vi "CIF_CIPC_String_Tag Update Test Cases.vi"() -> (0 "error out":errorcluster, 2 "status":string, 3 "pass":bool)   [LabVIEW 2021]
uses:
  CIFChannels/Typedef/Direction.ctl
  CIF_CIPC_Chn_String.lvclass
  D:/dev/Packages/CIF_Channels_Core/src/CIFChannels/CIFChannels.lvclass
  ChannelCommon/typedef/New FIFO Instance Response.ctl
  ChannelCommon/typedef/New FIFO Config.ctl
  ChannelCommon/typedef/FIFO Flags.ctl
  ChannelCommon/Utilities/Flatten FIFO Config.vi
  ChannelCommon/Utilities/Flatten FIFO Flags.vi
  <vilib>/CIF Foundation/CIF Utilities/DataTypes/Flatten Unflatten/Flatten U64.vi
  CIFChannels/CIFChannels.lvclass
  ChannelCommon/ChannelCommon.lvlib
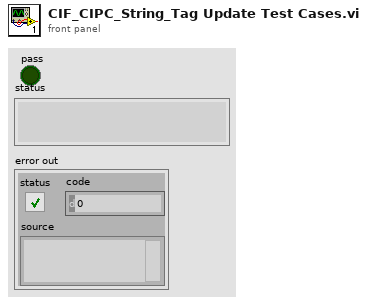
[diagram p1: front panel]
types:
  T1 = typedef "CIFChannels.lvclass/Direction.ctl" = enum16{"Publisher", "Subscriber"}
  T2 = typedef "ChannelCommon.lvlib/New FIFO Instance Response.ctl" = cluster{"Publisher":string, "Custom Data":u8[]}
  T3 = typedef "ChannelCommon.lvlib/New FIFO Config.ctl" = cluster{"Max Bytes/Msg":u64, "Max Msg/FIFO":u64, "FIFO Flags":T4}
  T4 = typedef "ChannelCommon.lvlib/FIFO Flags.ctl" = cluster{"Backpressure":bool}
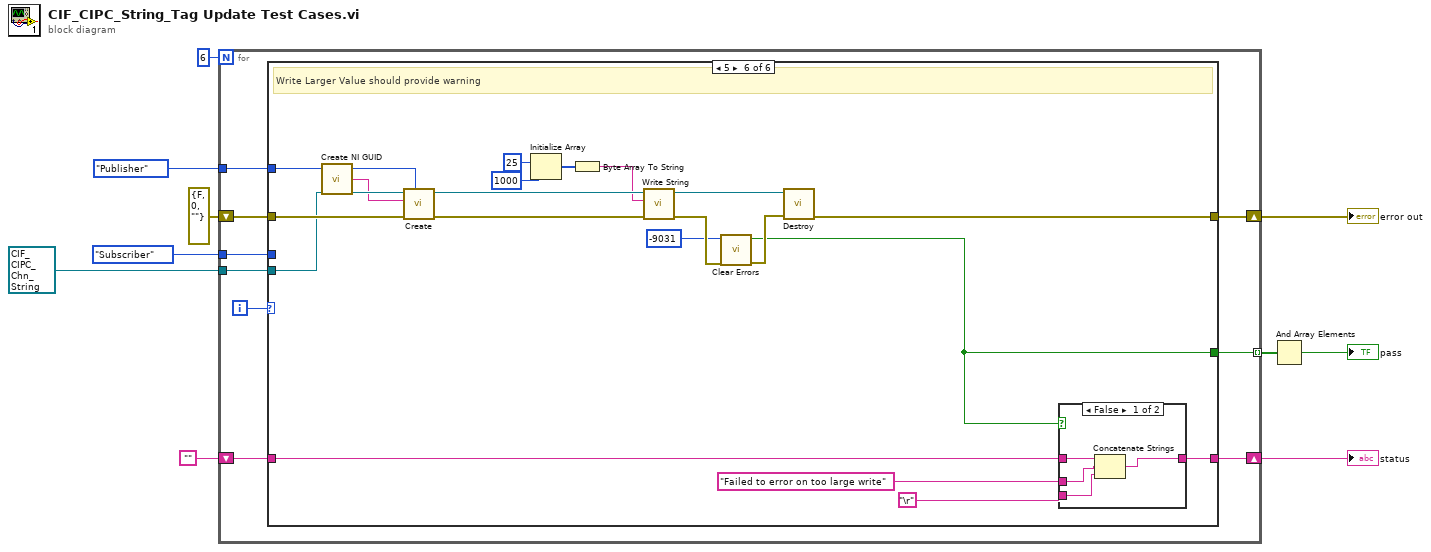
[diagram p0: block diagram]
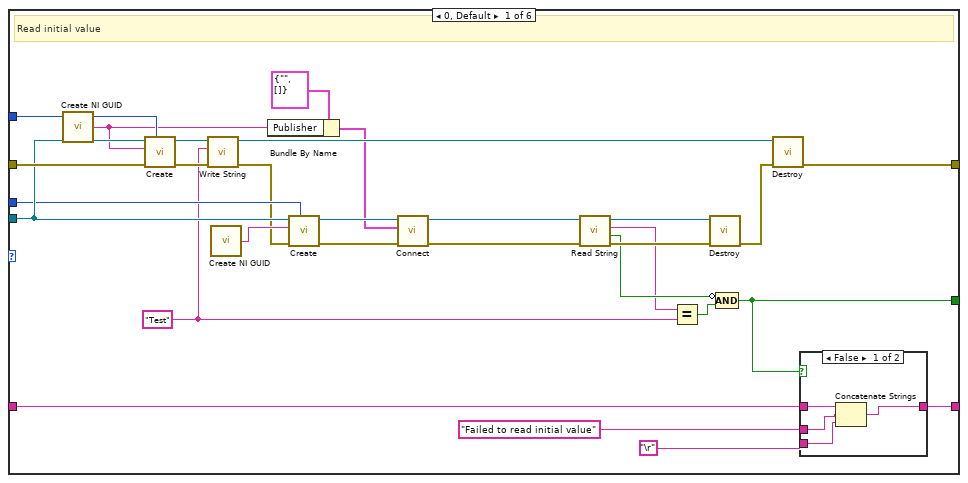
[diagram p2: hidden frame]
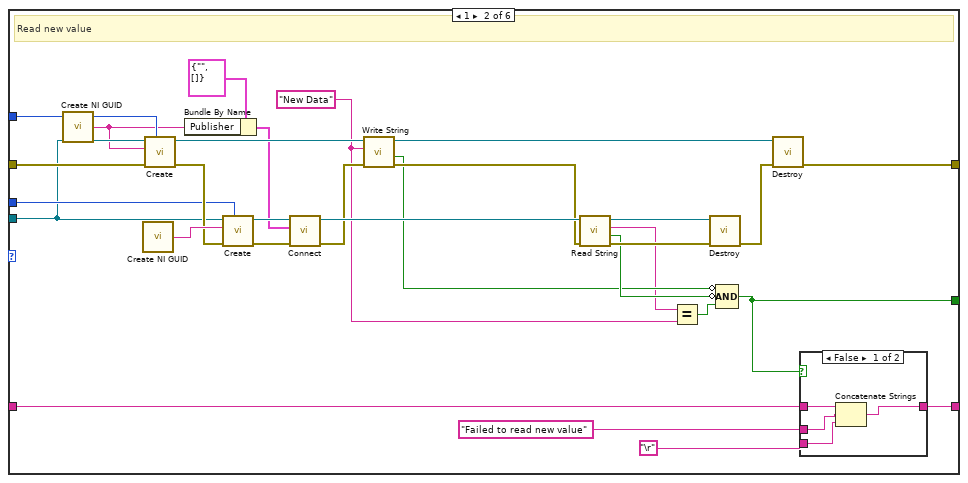
[diagram p4: hidden frame]
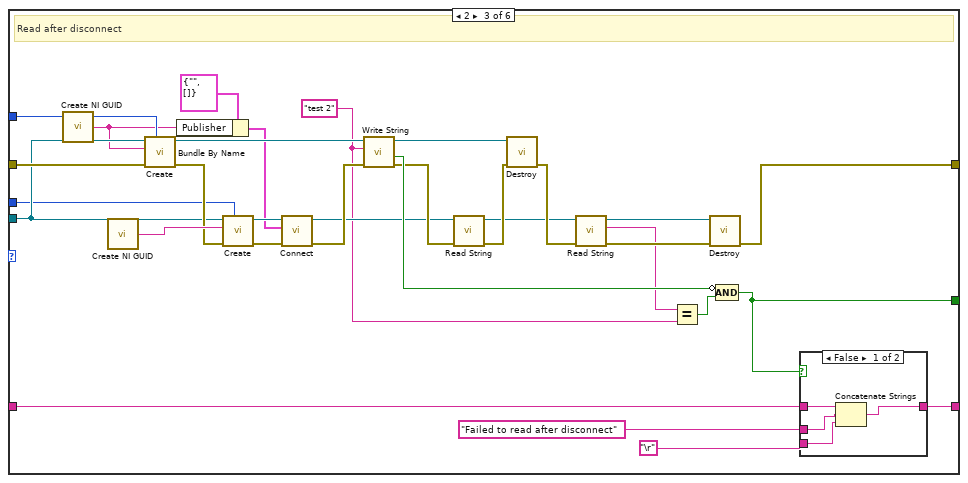
[diagram p6: hidden frame]
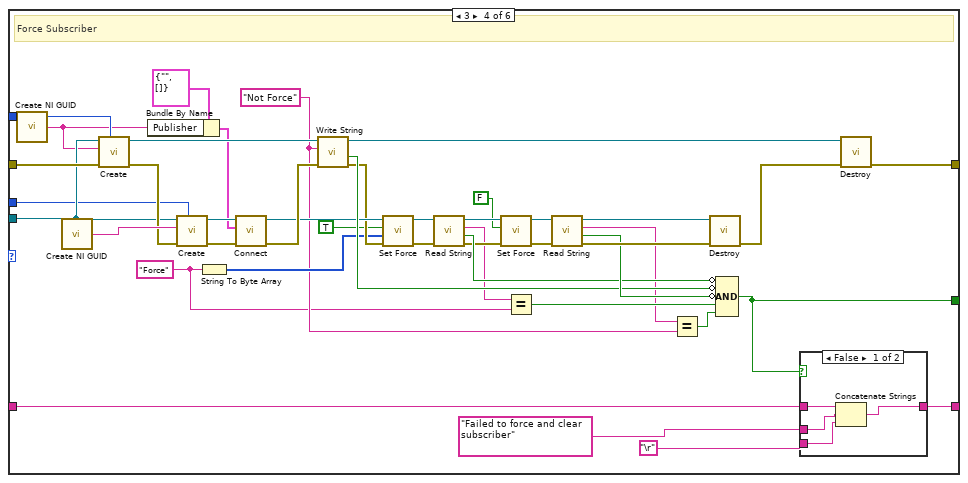
[diagram p8: hidden frame]
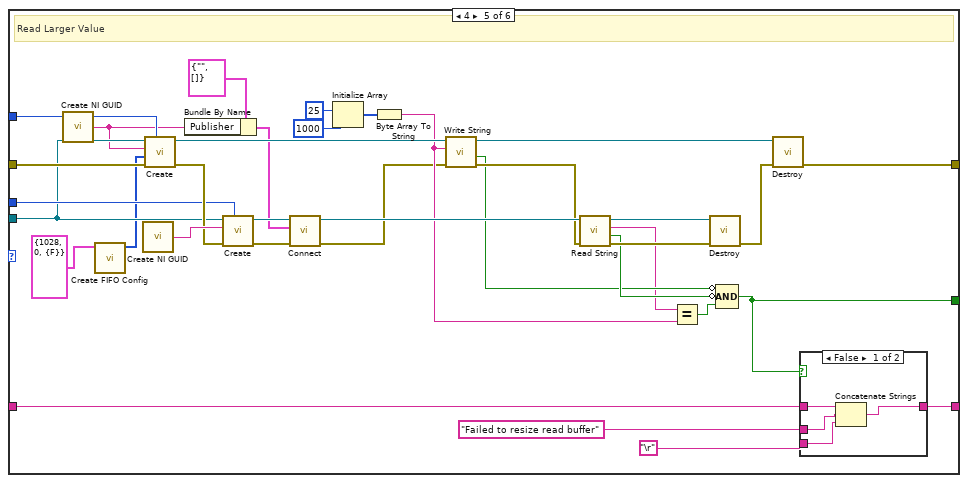
[diagram p10: hidden frame]
diagram:
  n1 = for {
    N: 6 -> [_]
    tunnel: [w19] -> w10 mode=indexing
    shift-right: [w17] -> w5
    shift-left: errorcluster {"status"=FALSE, "code"=0, "source"=""} ("error out") -> [w18]
    shift-right: [w14] -> w6
    shift-left: "" -> [w15]
    tunnel: refnum<class "CIF_CIPC_Chn_String.lvclass"> refnum ("CIF_CIPC_Chn_String.lvclass") -> [w13]
    tunnel: Direction."Publisher" ("Direction") -> [w12]
    tunnel: Direction."Subscriber" ("Direction") -> [w11]
    i -> [w16]
    n2 = case shown="5" w16 {
      tunnel: [w33 w68 w111 w158 w192 w213] -> w19
      tunnel: w18 -> [w44 w79 w115 w163 w203 w228]
      tunnel: [w35 w70 w105 w132 w194 w227] -> w17
      tunnel: w15 -> [w48 w83 w119 w167 w207 w232]
      tunnel: [w47 w82 w118 w166 w206 w231] -> w14
      tunnel: w13 -> [w30 w59 w100 w150 w184 w223]
      tunnel: w12 -> [w31 w61 w99 w149 w186 w224]
      tunnel: w11 -> [w29 w60 w98 w148 w185 _]
      frame 0, Default {
        w21 = "Test"
        # "Read initial value"
        n3 = call <vilib>:"Create NI GUID.vi"() -> ("NI GUID"=w23:string)
        n4 = call-dynamic "Create.vi"("Direction"=w31, "error in (no error)"=w44, "Name"=w23, "CIFTag in"=w30) -> ("error out"=w27:errorcluster, "CIFTag out"=w28:refnum<class "CIF_CIPC_Chn_String.lvclass">)  [unwired: 6 in]
        n5 = call-dynamic "Write String.vi"("error in (no error)"=w27, "Data"=w21, "CIFTag in"=w28) -> ("error out"=w25:errorcluster, "CIFTag out"=w26:refnum<class "CIF_CIPC_Chn_String.lvclass">)  [unwired: 6 in, 1 out]
        n6 = call <vilib>:"Create NI GUID.vi"() -> ("NI GUID"=w43:string)
        n7 = Bundle By Name(cluster=T2 {"Publisher"="", "Custom Data"=[]} ("Connection"), "Publisher"=w23) -> (w22:T2)
        n8 = call-dynamic "Create.vi"("Direction"=w29, "error in (no error)"=w25, "Name"=w43, "CIFTag in"=w30) -> ("error out"=w41:errorcluster, "CIFTag out"=w42:refnum<class "CIF_CIPC_Chn_String.lvclass">)  [unwired: 6 in]
        n9 = call-dynamic "Connect.vi"("error in (no error)"=w41, "Connection"=w22, "CIFTag in"=w42) -> ("error out"=w39:errorcluster, "CIFTag out"=w40:refnum<class "CIF_CIPC_Chn_String.lvclass">)  [unwired: 7 in]
        n10 = call-dynamic "Read String.vi"("error in (no error)"=w39, "CIFTag in"=w40) -> ("error out"=w37:errorcluster, "timed out?"=w32:bool, "Data"=w20:string, "CIFTag out"=w38:refnum<class "CIF_CIPC_Chn_String.lvclass">)  [unwired: 6 in]
        n11 = Equal?(x=w20, y=w21) -> (x = y?=w34:bool)
        n12 = call-dynamic "Destroy.vi"("error in (no error)"=w37, "CIFTag in"=w38) -> ("error out"=w36:errorcluster)  [unwired: 8 in, 1 out]
        n13 = Compound Arithmetic op=AND(invert w32, w34) -> (w33:bool)
        n14 = call-dynamic "Destroy.vi"("error in (no error)"=w36, "CIFTag in"=w26) -> ("error out"=w35:errorcluster)  [unwired: 8 in, 1 out]
        n15 = case shown="False" w33 {
          tunnel: w48 -> [w52 w53]
          tunnel: [w49 w53] -> w47
          tunnel: "Failed to read initial value" -> [w51 _]
          tunnel: "\r" -> [w50 _]
          frame False {
            n16 = Concatenate Strings(w52, w51, w50) -> (w49:string)
          }
          frame True {
          }
        }
      }
      frame 1 {
        w55 = "New Data" ("Data")
        # "Read new value"
        n17 = call <vilib>:"Create NI GUID.vi"() -> ("NI GUID"=w57:string)
        n18 = call <vilib>:"Create NI GUID.vi"() -> ("NI GUID"=w78:string)
        n19 = call-dynamic "Create.vi"("Direction"=w61, "error in (no error)"=w79, "Name"=w57, "CIFTag in"=w59) -> ("error out"=w77:errorcluster, "CIFTag out"=w66:refnum<class "CIF_CIPC_Chn_String.lvclass">)  [unwired: 6 in]
        n20 = Bundle By Name(cluster=T2 {"Publisher"="", "Custom Data"=[]} ("Connection"), "Publisher"=w57) -> (w56:T2)
        n21 = call-dynamic "Create.vi"("Direction"=w60, "error in (no error)"=w77, "Name"=w78, "CIFTag in"=w59) -> ("error out"=w75:errorcluster, "CIFTag out"=w76:refnum<class "CIF_CIPC_Chn_String.lvclass">)  [unwired: 6 in]
        n22 = call-dynamic "Connect.vi"("error in (no error)"=w75, "Connection"=w56, "CIFTag in"=w76) -> ("error out"=w65:errorcluster, "CIFTag out"=w74:refnum<class "CIF_CIPC_Chn_String.lvclass">)  [unwired: 7 in]
        n23 = call-dynamic "Write String.vi"("error in (no error)"=w65, "Data"=w55, "CIFTag in"=w66) -> ("error out"=w64:errorcluster, "timed out?"=w62:bool, "CIFTag out"=w63:refnum<class "CIF_CIPC_Chn_String.lvclass">)  [unwired: 6 in]
        n24 = call-dynamic "Read String.vi"("error in (no error)"=w64, "CIFTag in"=w74) -> ("error out"=w72:errorcluster, "timed out?"=w67:bool, "Data"=w54:string, "CIFTag out"=w73:refnum<class "CIF_CIPC_Chn_String.lvclass">)  [unwired: 6 in]
        n25 = Equal?(x=w54, y=w55) -> (x = y?=w69:bool)
        n26 = call-dynamic "Destroy.vi"("error in (no error)"=w72, "CIFTag in"=w73) -> ("error out"=w71:errorcluster)  [unwired: 8 in, 1 out]
        n27 = Compound Arithmetic op=AND(invert w62, invert w67, w69) -> (w68:bool)
        n28 = call-dynamic "Destroy.vi"("error in (no error)"=w71, "CIFTag in"=w63) -> ("error out"=w70:errorcluster)  [unwired: 8 in, 1 out]
        n29 = case shown="False" w68 {
          tunnel: w83 -> [w87 w88]
          tunnel: [w84 w88] -> w82
          tunnel: "Failed to read new value" -> [w86 _]
          tunnel: "\r" -> [w85 _]
          frame False {
            n30 = Concatenate Strings(w87, w86, w85) -> (w84:string)
          }
          frame True {
          }
        }
      }
      frame 2 {
        w90 = "test 2" ("Data")
        # "Read after disconnect"
        n31 = call <vilib>:"Create NI GUID.vi"() -> ("NI GUID"=w92:string)
        n32 = call <vilib>:"Create NI GUID.vi"() -> ("NI GUID"=w114:string)
        n33 = call-dynamic "Create.vi"("Direction"=w99, "error in (no error)"=w115, "Name"=w92, "CIFTag in"=w100) -> ("error out"=w113:errorcluster, "CIFTag out"=w110:refnum<class "CIF_CIPC_Chn_String.lvclass">)  [unwired: 6 in]
        n34 = Bundle By Name(cluster=T2 {"Publisher"="", "Custom Data"=[]} ("Connection"), "Publisher"=w92) -> (w91:T2)
        n35 = call-dynamic "Create.vi"("Direction"=w98, "error in (no error)"=w113, "Name"=w114, "CIFTag in"=w100) -> ("error out"=w103:errorcluster, "CIFTag out"=w104:refnum<class "CIF_CIPC_Chn_String.lvclass">)  [unwired: 6 in]
        n36 = call-dynamic "Connect.vi"("error in (no error)"=w103, "Connection"=w91, "CIFTag in"=w104) -> ("error out"=w102:errorcluster, "CIFTag out"=w101:refnum<class "CIF_CIPC_Chn_String.lvclass">)  [unwired: 7 in]
        n37 = call-dynamic "Write String.vi"("error in (no error)"=w102, "Data"=w90, "CIFTag in"=w110) -> ("error out"=w108:errorcluster, "timed out?"=w109:bool, "CIFTag out"=w107:refnum<class "CIF_CIPC_Chn_String.lvclass">)  [unwired: 6 in]
        n38 = call-dynamic "Read String.vi"("error in (no error)"=w108, "CIFTag in"=w101) -> ("error out"=w106:errorcluster, "CIFTag out"=w96:refnum<class "CIF_CIPC_Chn_String.lvclass">)  [unwired: 6 in, 2 out]
        n39 = call-dynamic "Destroy.vi"("error in (no error)"=w106, "CIFTag in"=w107) -> ("error out"=w97:errorcluster)  [unwired: 8 in, 1 out]
        n40 = call-dynamic "Read String.vi"("error in (no error)"=w97, "CIFTag in"=w96) -> ("error out"=w95:errorcluster, "Data"=w89:string, "CIFTag out"=w94:refnum<class "CIF_CIPC_Chn_String.lvclass">)  [unwired: 6 in, 1 out]
        n41 = Equal?(x=w89, y=w90) -> (x = y?=w112:bool)
        n42 = call-dynamic "Destroy.vi"("error in (no error)"=w95, "CIFTag in"=w94) -> ("error out"=w105:errorcluster)  [unwired: 8 in, 1 out]
        n43 = Compound Arithmetic op=AND(invert w109, w112) -> (w111:bool)
        n44 = case shown="False" w111 {
          tunnel: w119 -> [w123 w124]
          tunnel: [w120 w124] -> w118
          tunnel: "Failed to read after disconnect" -> [w122 _]
          tunnel: "\r" -> [w121 _]
          frame False {
            n45 = Concatenate Strings(w123, w122, w121) -> (w120:string)
          }
          frame True {
          }
        }
      }
      frame 3 {
        w125 = "Force" ("string")
        w128 = "Not Force" ("Data")
        # "Force Subscriber"
        n46 = call <vilib>:"Create NI GUID.vi"() -> ("NI GUID"=w130:string)
        n47 = call <vilib>:"Create NI GUID.vi"() -> ("NI GUID"=w162:string)
        n48 = call-dynamic "Create.vi"("Direction"=w149, "error in (no error)"=w163, "Name"=w130, "CIFTag in"=w150) -> ("error out"=w161:errorcluster, "CIFTag out"=w156:refnum<class "CIF_CIPC_Chn_String.lvclass">)  [unwired: 6 in]
        n49 = Bundle By Name(cluster=T2 {"Publisher"="", "Custom Data"=[]} ("Connection"), "Publisher"=w130) -> (w129:T2)
        n50 = call-dynamic "Create.vi"("Direction"=w148, "error in (no error)"=w161, "Name"=w162, "CIFTag in"=w150) -> ("error out"=w152:errorcluster, "CIFTag out"=w153:refnum<class "CIF_CIPC_Chn_String.lvclass">)  [unwired: 6 in]
        n51 = String To Byte Array(string=w125) -> (unsigned byte array=w145:u8[])
        n52 = call-dynamic "Connect.vi"("error in (no error)"=w152, "Connection"=w129, "CIFTag in"=w153) -> ("error out"=w151:errorcluster, "CIFTag out"=w147:refnum<class "CIF_CIPC_Chn_String.lvclass">)  [unwired: 7 in]
        n53 = call-dynamic "Write String.vi"("error in (no error)"=w151, "Data"=w128, "CIFTag in"=w156) -> ("error out"=w146:errorcluster, "timed out?"=w155:bool, "CIFTag out"=w154:refnum<class "CIF_CIPC_Chn_String.lvclass">)  [unwired: 6 in]
        n54 = call "Set Force.vi"("error in (no error)"=w146, "Force Data"=w145, "Force Active"=TRUE, "CIFChannels in"=w147) -> ("error out"=w142:errorcluster, "CIFChannels out"=w143:refnum<class "CIF_CIPC_Chn_String.lvclass">)  [unwired: 6 in]
        n55 = call-dynamic "Read String.vi"("error in (no error)"=w142, "CIFTag in"=w143) -> ("error out"=w137:errorcluster, "timed out?"=w141:bool, "Data"=w126:string, "CIFTag out"=w138:refnum<class "CIF_CIPC_Chn_String.lvclass">)  [unwired: 6 in]
        n56 = call "Set Force.vi"("error in (no error)"=w137, "Force Active"=FALSE, "CIFChannels in"=w138) -> ("error out"=w136:errorcluster, "CIFChannels out"=w135:refnum<class "CIF_CIPC_Chn_String.lvclass">)  [unwired: 7 in]
        n57 = Equal?(x=w126, y=w125) -> (x = y?=w139:bool)
        n58 = call-dynamic "Read String.vi"("error in (no error)"=w136, "CIFTag in"=w135) -> ("error out"=w159:errorcluster, "timed out?"=w157:bool, "Data"=w127:string, "CIFTag out"=w160:refnum<class "CIF_CIPC_Chn_String.lvclass">)  [unwired: 6 in]
        n59 = Equal?(x=w127, y=w128) -> (x = y?=w140:bool)
        n60 = call-dynamic "Destroy.vi"("error in (no error)"=w159, "CIFTag in"=w160) -> ("error out"=w133:errorcluster)  [unwired: 8 in, 1 out]
        n61 = Compound Arithmetic op=AND(invert w141, invert w155, invert w157, w139, w140) -> (w158:bool)
        n62 = case shown="False" w158 {
          tunnel: w167 -> [w171 w172]
          tunnel: [w168 w172] -> w166
          tunnel: "Failed to force and clear subscriber" -> [w170 _]
          tunnel: "\r" -> [w169 _]
          frame False {
            n63 = Concatenate Strings(w171, w170, w169) -> (w168:string)
          }
          frame True {
          }
        }
        n64 = call-dynamic "Destroy.vi"("error in (no error)"=w133, "CIFTag in"=w154) -> ("error out"=w132:errorcluster)  [unwired: 8 in, 1 out]
      }
      frame 4 {
        # "Read Larger Value"
        n65 = call <vilib>:"Create NI GUID.vi"() -> ("NI GUID"=w182:string)
        n66 = call "Create FIFO Config.vi"("New FIFO Config"=T3 {"Max Bytes/Msg"=1028, "Max Msg/FIFO"=0, "FIFO Flags"={"Backpressure"=FALSE}}) -> ("Flattened FIFO Config"=w179:u8[])  [unwired: 10 in]
        n67 = call <vilib>:"Create NI GUID.vi"() -> ("NI GUID"=w202:string)
        n68 = call-dynamic "Create.vi"("Direction"=w186, "error in (no error)"=w203, "Custom Config Data"=w179, "Name"=w182, "CIFTag in"=w184) -> ("error out"=w201:errorcluster, "CIFTag out"=w190:refnum<class "CIF_CIPC_Chn_String.lvclass">)  [unwired: 5 in]
        n69 = Bundle By Name(cluster=T2 {"Publisher"="", "Custom Data"=[]} ("Connection"), "Publisher"=w182) -> (w181:T2)
        n70 = call-dynamic "Create.vi"("Direction"=w185, "error in (no error)"=w201, "Name"=w202, "CIFTag in"=w184) -> ("error out"=w199:errorcluster, "CIFTag out"=w200:refnum<class "CIF_CIPC_Chn_String.lvclass">)  [unwired: 6 in]
        n71 = call-dynamic "Connect.vi"("error in (no error)"=w199, "Connection"=w181, "CIFTag in"=w200) -> ("error out"=w173:errorcluster, "CIFTag out"=w198:refnum<class "CIF_CIPC_Chn_String.lvclass">)  [unwired: 7 in]
        n72 = Initialize Array(u8 25 ("element"), 1000 ("dimension size")) -> (w175:u8[])
        n73 = Byte Array To String(unsigned byte array=w175) -> (string=w174:string)
        n74 = call-dynamic "Write String.vi"("error in (no error)"=w173, "Data"=w174, "CIFTag in"=w190) -> ("error out"=w189:errorcluster, "timed out?"=w187:bool, "CIFTag out"=w188:refnum<class "CIF_CIPC_Chn_String.lvclass">)  [unwired: 6 in]
        n75 = call-dynamic "Read String.vi"("error in (no error)"=w189, "CIFTag in"=w198) -> ("error out"=w196:errorcluster, "timed out?"=w191:bool, "Data"=w180:string, "CIFTag out"=w197:refnum<class "CIF_CIPC_Chn_String.lvclass">)  [unwired: 6 in]
        n76 = Equal?(x=w180, y=w174) -> (x = y?=w193:bool)
        n77 = call-dynamic "Destroy.vi"("error in (no error)"=w196, "CIFTag in"=w197) -> ("error out"=w195:errorcluster)  [unwired: 8 in, 1 out]
        n78 = Compound Arithmetic op=AND(invert w187, invert w191, w193) -> (w192:bool)
        n79 = call-dynamic "Destroy.vi"("error in (no error)"=w195, "CIFTag in"=w188) -> ("error out"=w194:errorcluster)  [unwired: 8 in, 1 out]
        n80 = case shown="False" w192 {
          tunnel: w207 -> [w211 w212]
          tunnel: [w208 w212] -> w206
          tunnel: "Failed to resize read buffer" -> [w210 _]
          tunnel: "\r" -> [w209 _]
          frame False {
            n81 = Concatenate Strings(w211, w210, w209) -> (w208:string)
          }
          frame True {
          }
        }
      }
      frame 5 {
        # "Write Larger Value should provide warning"
        n82 = call <vilib>:"Create NI GUID.vi"() -> ("NI GUID"=w222:string)
        n83 = call-dynamic "Create.vi"("Direction"=w224, "error in (no error)"=w228, "Name"=w222, "CIFTag in"=w223) -> ("error out"=w217:errorcluster, "CIFTag out"=w226:refnum<class "CIF_CIPC_Chn_String.lvclass">)  [unwired: 6 in]
        n84 = Initialize Array(u8 25 ("element"), 1000 ("dimension size")) -> (w219:u8[])
        n85 = Byte Array To String(unsigned byte array=w219) -> (string=w218:string)
        n86 = call-dynamic "Write String.vi"("error in (no error)"=w217, "Data"=w218, "CIFTag in"=w226) -> ("error out"=w216:errorcluster, "CIFTag out"=w225:refnum<class "CIF_CIPC_Chn_String.lvclass">)  [unwired: 6 in, 1 out]
        n87 = call <vilib>:"Clear Errors.vi"("error in (no error)"=w216, "specific error code to clear (0: all)"=-9031) -> ("error out"=w215:errorcluster, "specific error cleared?"=w213:bool)  [unwired: 4 in]
        n88 = call-dynamic "Destroy.vi"("error in (no error)"=w215, "CIFTag in"=w225) -> ("error out"=w227:errorcluster)  [unwired: 8 in, 1 out]
        n89 = case shown="False" w213 {
          tunnel: w232 -> [w236 w237]
          tunnel: [w233 w237] -> w231
          tunnel: "Failed to error on too large write" -> [w235 _]
          tunnel: "\r" -> [w234 _]
          frame False {
            n90 = Concatenate Strings(w236, w235, w234) -> (w233:string)
          }
          frame True {
          }
        }
      }
    }
  }
  "error out" <- w5
  "status" <- w6
  n91 = And Array Elements(Boolean array=w10) -> (logical AND=→"pass":bool)
